vi "Convert_StringToBool.vi"(9 "node text":string) -> (1 "bool":bool)   [LabVIEW 2010, in "Pansino_XML_Read.lvlib"]
uses:
  Pansino_XML_Read.lvlib
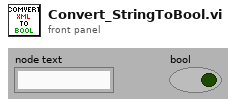
[diagram p1: front panel]
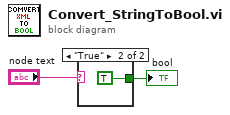
[diagram p0: block diagram]
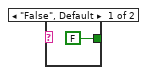
[diagram p2: hidden frame]
diagram:
  n1 = case shown="\"True\"" "node text" {
    tunnel: [FALSE ("握手") TRUE ("握手")] -> w1
    frame "False", Default {
    }
    frame "True" {
    }
  }
  "bool" <- w1
